vi "Set Index.vi"(8 "error in (no error)":errorcluster, 10 "Index":i32, 11 "Abs_Waveform in":refnum<class "Abs_Waveform.lvclass">) -> (0 "error out":errorcluster, 3 "Abs_Waveform out":refnum<class "Abs_Waveform.lvclass">)   [LabVIEW 2021, in "Abs_Waveform.lvclass"]
uses:
  Abs_Waveform.lvclass
  Abs_Waveform.lvclass/Abs_Waveform.ctl
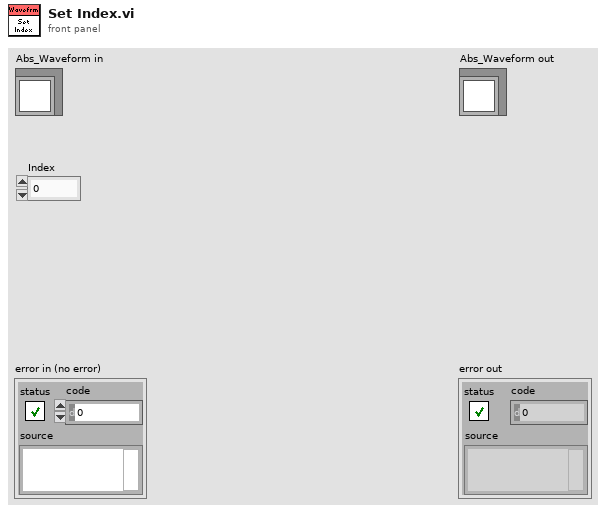
[diagram p1: front panel]
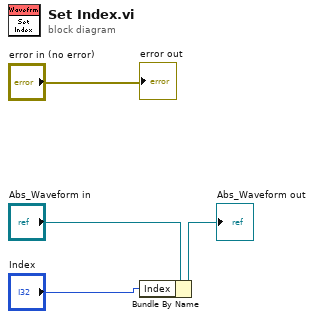
[diagram p0: block diagram]
diagram:
  n1 = Bundle By Name(cluster="Abs_Waveform in", "Index"="Index") -> (→"Abs_Waveform out":refnum<class "Abs_Waveform.lvclass">)
  "error out" <- "error in (no error)"
